vi "Items Read.vi"(4 "error in (no error)":errorcluster, 6 "Container State":T2, 7 "Display State In":T1) -> (0 "error out":errorcluster, 2 "Value":string[](array[string]), 3 "Display State Out":T1)   [LabVIEW 2015, in "Trigger.xctl"]
uses:
  Trigger.xctl
  <vilib>/_xctls/Container State.ctl
  <vilib>/_xctls/XControlSupport.lvlib
  State.ctl
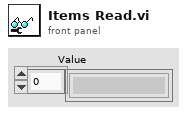
[diagram p1: front panel]
types:
  T1 = typedef "Trigger.xctl/State.ctl" = cluster{"Name":string, "Strings and Formats":cluster{"Items":string[], "Formats":string[]}}
  T2 = typedef "XControlSupport.lvlib/Container State.ctl" = cluster{"Indicator?":bool, "Run Mode?":bool, " Refnum":refnum<vi>}
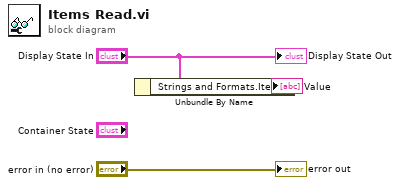
[diagram p0: block diagram]
diagram:
  n1 = Unbundle By Name("Display State In") -> ("Strings and Formats.Items"=→"Value":string[])
  "error out" <- "error in (no error)"
  "Display State Out" <- "Display State In"
